vi "DRAM_latency_test.vi"() -> ()   [LabVIEW 2024]
uses:
  <vilib>/rvi/Memory/Memory_Emulation/nirvimemoryFastEmulation.vi
  <vilib>/rvi/Memory/Memory_Emulation/nirvimemoryEmulation.vi
  <vilib>/rvi/Emulation/niFpgaEmulationIsFPGAContextNoSignature.vi
  <vilib>/rvi/DataTransferAndStorage/Container/Common/niFpgaContainerGetUniqueNameForEmu.vi
  <vilib>/rvi/Emulation/niFpgaProcessEmulError.vi
  <vilib>/rvi/Emulation/niFpgaSctlEmulationGetInTimedLoop.vi
  <vilib>/rvi/errors/nirviReportUnexpectedCaseInternalError (U32).vi
  <vilib>/rvi/DataTransferAndStorage/Container/XNode/niFpgaContainer.xnode
panel:
  out "data6":i16
  out "data5":i16
  out "data4":i16
  out "data3":i16
  out "data2":i16
  out "data1":i16
  out "data0":i16
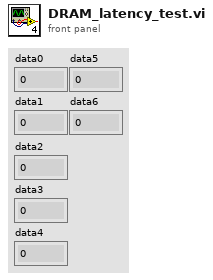
[diagram p1: front panel]
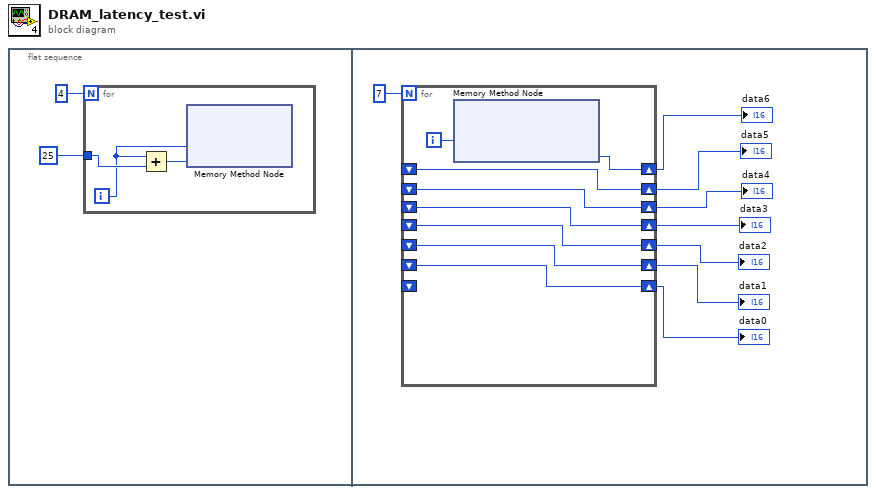
[diagram p0: block diagram]
diagram:
  n1 = flat-sequence {
    frame #0 {
      n2 = for {
        N: 4 -> [_]
        tunnel: i16 25 -> [w5]
        i -> [w4]
        n3 = Add(x=w4, y=w5) -> (x+y=w3:i32)
        n4 = xnode ("Memory Method Node")("Address"=w4, "Data"=w3) -> ()  [unwired: 1 in, 1 out]
      }
    }
    frame #1 {
      n5 = for {
        N: 7 -> [_]
        shift-right: [w20] -> w6
        shift-left: _ -> [w19]
        shift-right: [w19] -> w7
        shift-left: _ -> [w18]
        shift-right: [w18] -> w8
        shift-left: _ -> [w17]
        shift-right: [w17] -> w9
        shift-left: _ -> [w16]
        shift-right: [w16] -> w10
        shift-left: _ -> [w15]
        shift-right: [w15] -> w11
        shift-left: _ -> [w14]
        shift-right: [w14] -> w12
        shift-left: _ -> [_]
        i -> [w21]
        n6 = xnode ("Memory Method Node")("Address"=w21) -> ("Data"=w20:i16)  [unwired: 1 in, 1 out]
      }
      "data0" <- w12
      "data1" <- w11
      "data2" <- w10
      "data3" <- w9
      "data4" <- w8
      "data5" <- w7
      "data6" <- w6
    }
  }
